vi "priv_GetAllPanesControls.vi"(8 "error in (no error)":errorcluster, 11 "UI_Actor in":refnum<class "UI_Actor.lvclass">) -> (0 "error out":errorcluster, 2 "Controls[]":refnum<vi>[](array[refnum]), 3 "UI_Actor out":refnum<class "UI_Actor.lvclass">)   [LabVIEW 2020, in "UI_Actor.lvlib" / "UI_Actor.lvclass"]
uses:
  UI_Actor.lvclass
  UI_Actor.lvclass/UI_Actor.ctl
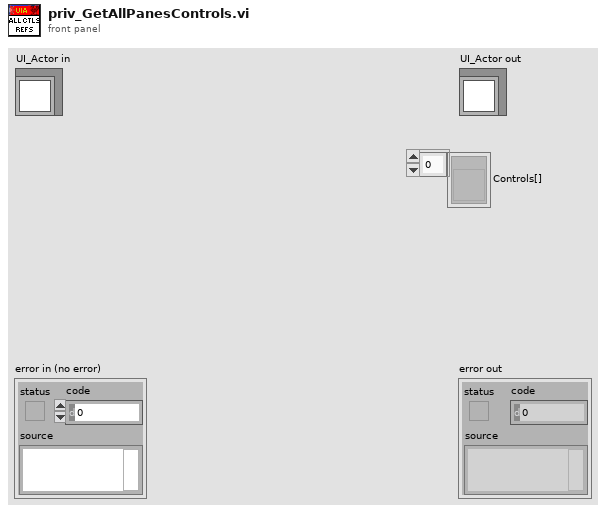
[diagram p1: front panel]
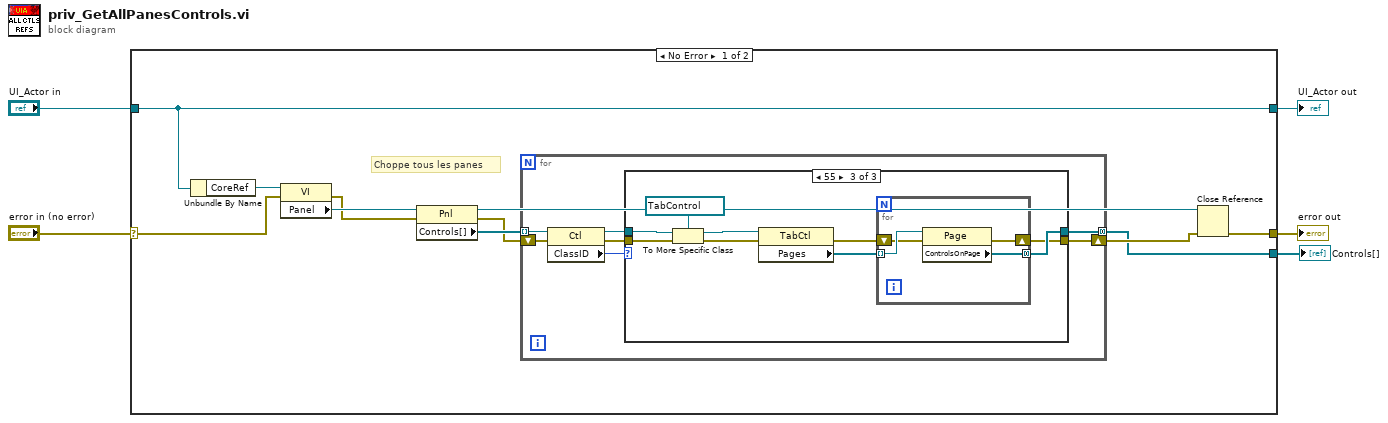
[diagram p0: block diagram]
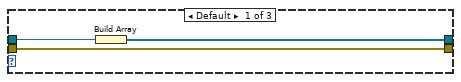
[diagram p2: hidden frame]
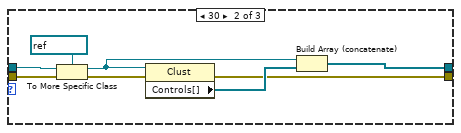
[diagram p3: hidden frame]
diagram:
  n1 = case shown="No Error" "error in (no error)" {
    selector: "error in (no error)" -> [w9 w49]
    tunnel: [w11 w49] -> w4
    tunnel: [w14 w48] -> w2
    tunnel: "UI_Actor in" -> [w14 w48]
    tunnel: [w8 _] -> w1
    frame No Error {
      # "Choppe tous les panes"
      n2 = Unbundle By Name(w14) -> ("CoreRef"=w16:refnum<vi>)
      n3 = property class="VI"(reference=w16, error in=w9) -> (error out=w10:errorcluster, "Panel"=w15:refnum<vi>)  [unwired: 1 out]
      n4 = property class="Pnl"(reference=w15, error in=w10) -> (reference out=w13:refnum<vi>, error out=w6:errorcluster, "Controls[]"=w7:refnum<vi>[])
      n5 = for {
        tunnel: w7 -> [w23] mode=indexing
        shift-right: [w18] -> w12
        shift-left: w6 -> [w22]
        tunnel: [w19] -> w8 mode=concatenating
        n6 = property class="Ctl"(reference=w23, error in=w22) -> (reference out=w20:refnum<vi>, error out=w17:errorcluster, "ClassID"=w21:u32)
        n7 = case shown="55" w21 {
          tunnel: [w25 w28 w36] -> w19
          tunnel: w20 -> [w26 w33 w42]
          tunnel: [w24 w29 w35] -> w18
          tunnel: w17 -> [w24 w34 w43]
          frame Default {
            n8 = Build Array(w26) -> (w25:refnum<vi>[])
          }
          frame 30 {
            n9 = To More Specific Class(target class=refnum<vi> refnum ("Cluster"), reference=w33, error in=w34) -> (specific class reference=w27:refnum<vi>, error out=w31:errorcluster)
            n10 = property class="Clust"(reference=w27, error in=w31) -> (error out=w29:errorcluster, "Controls[]"=w30:refnum<vi>[])  [unwired: 1 out]
            n11 = Build Array (concatenate)(w27, w30) -> (w28:refnum<vi>[])
          }
          frame 55 {
            n12 = To More Specific Class(target class=refnum<vi> refnum ("Tab Control"), reference=w42, error in=w43) -> (specific class reference=w41:refnum<vi>, error out=w40:errorcluster)
            n13 = property class="TabCtl"(reference=w41, error in=w40) -> (error out=w37:errorcluster, "Pages"=w38:refnum<vi>[])  [unwired: 1 out]
            n14 = for {
              tunnel: w38 -> [w47] mode=indexing
              shift-right: [w45] -> w35
              shift-left: w37 -> [w46]
              tunnel: [w44] -> w36 mode=concatenating
              n15 = property class="Page"(reference=w47, error in=w46) -> (error out=w45:errorcluster, "ControlsOnPage"=w44:refnum<vi>[])  [unwired: 1 out]
            }
          }
        }
      }
      n16 = Close Reference(reference=w13, error in (no error)=w12) -> (error out=w11:errorcluster)
    }
    frame Error {
    }
  }
  "error out" <- w4
  "UI_Actor out" <- w2
  "Controls[]" <- w1
